vi "Write Terminal.vi"(8 "Error In":errorcluster, 10 "Terminal":T1, 11 "Channel In":refnum<class "Channel.lvclass">) -> (0 "Error Out":errorcluster, 3 "Channel Out":refnum<class "Channel.lvclass">)   [LabVIEW 2021, in "Field_RnD_Services_LIBSSH2_Toolkit.lvlib" / "Channel.lvclass"]
doc: "Sets the kind of terminal to use with a Shell-style channel."
uses:
  Channel.lvclass
  Session/Session.lvclass
  Field_RnD_Services_LIBSSH2_Toolkit.lvlib
  Type Definitions/Terminals.ctl
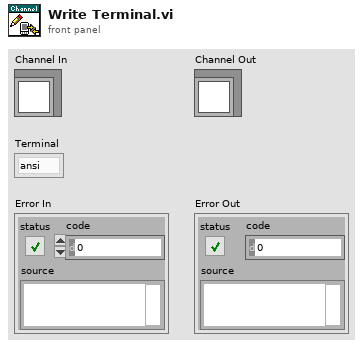
[diagram p1: front panel]
types:
  T1 = typedef "Field_RnD_Services_LIBSSH2_Toolkit.lvlib/Channel.lvclass/Terminals.ctl" = enum16{"ansi", "dump", "linux", "rxvt", "screen", "sun", "vt100", "vt102", "vt220", "vt52", "xterm"}
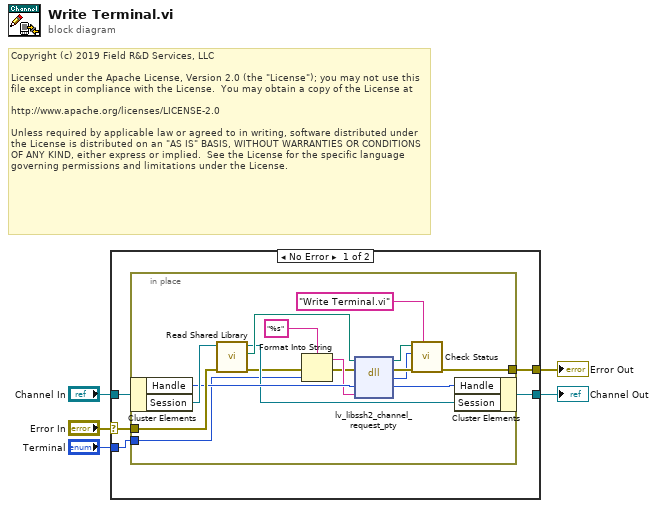
[diagram p0: block diagram]
diagram:
  # "Copyright (c) 2019 Field R&D Services, LLC\n\nLicensed under the Apache License, Version 2.0 (the \"License\"); you may not use this file except in compliance with the License.  You may obtain a copy of the License at\n\nhttp://www.apache.org/licenses/LICENSE-2.0\n\nUnless required by applicable law or agreed to in writing, software distributed under the License is distributed on an \"AS IS\" BASIS, WITHOUT WARRANTIES OR CONDITIONS OF ANY KIND, either express or implied.  See the License for the specific language governing permissions and limitations under the License."
  n1 = case shown="No Error" "Error In" {
    selector: "Error In" -> [w8 w28]
    tunnel: [w7 w28] -> w4
    tunnel: "Channel In" -> [w10 w27]
    tunnel: [w9 w27] -> w2
    tunnel: "Terminal" -> [w6 _]
    frame No Error {
      n2 = in-place {
        in-place-border: w8 -> [w24]
        in-place-border: [w20] -> w7
        in-place-border: w6 -> [w15]
        n3 = in-place-cluster #1(w10) -> ("Handle"=w19:u64, "Session"=w26:refnum<class "Session.lvclass">)
        n4 = call "Read Shared Library.vi"("Error In"=w24, "Session In"=w26) -> ("Erorr Out"=w16:errorcluster, "libssh2lv Shared Library"=w25:path, "Session Out"=w17:refnum<class "Session.lvclass">)  [unwired: 7 in]
        n5 = Format Into String(format string="%s", error in=w16, w15) -> (resulting string=w13:string, error out=w12:errorcluster)  [unwired: 1 in]
        n6 = dll-call lib="libssh2lv.*" fn="lv_libssh2_channel_request_pty"(path in=w25, error in=w12, "handle"=w19, "terminal"=w13) -> (path out=w22:path, error out=w23:errorcluster, "status"=w21:i32, "handle"=w18:u64)  [unwired: 2 in]
        n7 = call "Check Status.vi"("Source (\"\")"="Write Terminal.vi" ("Source (\"\")"), "Error In"=w23, "Status"=w21, "libssh2lv Shared Library In"=w22) -> ("Error Out"=w20:errorcluster)  [unwired: 6 in, 1 out]
        n8 = in-place-cluster #1("Handle"=w18, "Session"=w17) -> (w9:refnum<class "Channel.lvclass">)
      }
    }
    frame Error {
    }
  }
  "Error Out" <- w4
  "Channel Out" <- w2
